vi "set_stage_and_electrode_init.vi"(9 "electrodes reference":refnum<vi>, 10 "Process list":T1, 11 "instrument config":T2) -> ()   [LabVIEW 2014]
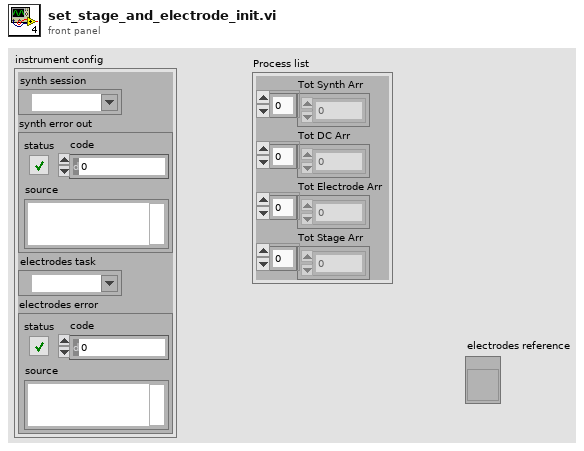
[diagram p1: front panel]
types:
  T1 = cluster{"Tot Synth Arr":dbl[], "Tot DC Arr":dbl[], "Tot Electrode Arr":dbl[], "Tot Stage Arr":dbl[]}
  T2 = cluster{"synth session":refnum<visa-resource-name>, "synth error out":errorcluster, "electrodes task":refnum<k21>, "electrodes error":errorcluster}
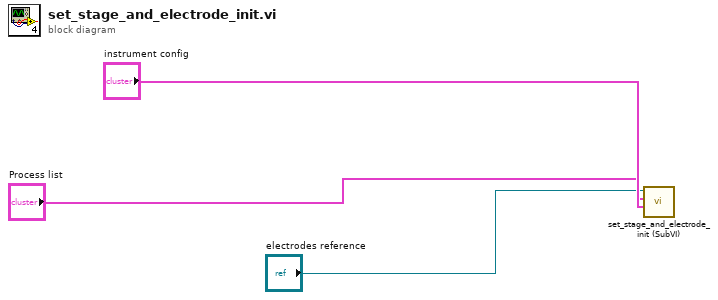
[diagram p0: block diagram]
diagram:
  n1 = call "set_stage_and_electrode_init (SubVI).vi"("instrument config"="instrument config", "Process list"="Process list", "Cluster in"="electrodes reference") -> ()  [unwired: 9 in]
